vi "Read GoToNearBallPlacementSkill.vi"(8 "error in (no error)":errorcluster, 11 "Skillbook in":refnum<class "Skillbook.lvclass">) -> (0 "error out":errorcluster, 2 "GoToNearBallPlacementSkill":refnum<class "GoToNearBallPlacementSkill.lvclass">, 3 "Skillbook out":refnum<class "Skillbook.lvclass">)   [LabVIEW 2023, in "Skillbook.lvclass"]
uses:
  Skillbook.lvclass
  GoToNearBallPlacementSkill_class/GoToNearBallPlacementSkill.lvclass
  Skillbook.lvclass/Skillbook.ctl
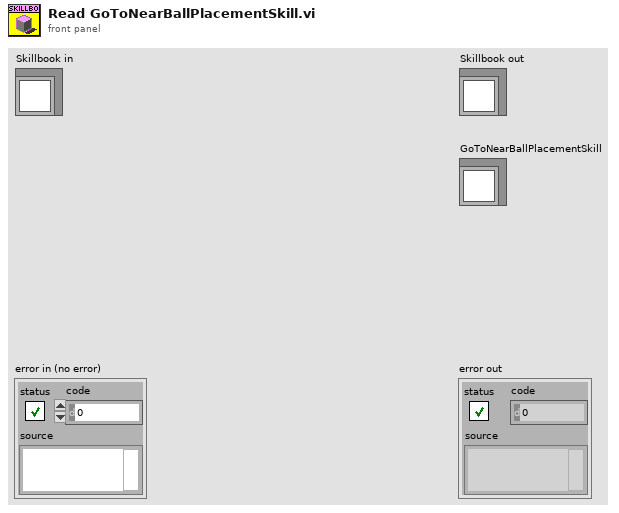
[diagram p1: front panel]
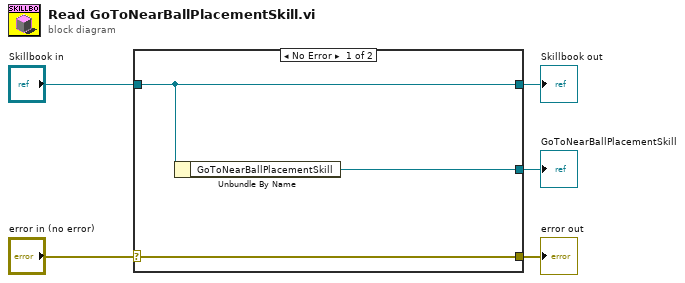
[diagram p0: block diagram]
diagram:
  n1 = case shown="No Error" "error in (no error)" {
    selector: "error in (no error)" -> [w8 w9]
    tunnel: [w8 w9] -> w4
    tunnel: [w7 w10] -> w2
    tunnel: "Skillbook in" -> [w7 w10]
    tunnel: [w6 _] -> w1
    frame No Error {
      n2 = Unbundle By Name(w7) -> ("GoToNearBallPlacementSkill"=w6:refnum<class "GoToNearBallPlacementSkill.lvclass">)
    }
    frame Error {
    }
  }
  "error out" <- w4
  "Skillbook out" <- w2
  "GoToNearBallPlacementSkill" <- w1
